vi "Butterfly_Resitance w_SMU.vi"(0 "Semiconductor Module Context":T3, 1 "script name":string="Cmax", 2 "SMU Settings":T2={"Level"=0.01, "Level Range"=0.1, "Limit"=1.0, "Limit Range"=6.0, "Sense"=0} {"Sense" items=["Local"=1008, "Remote"=1009]}, 5 "Pins":string[](array[string])=["RF"], 7 "HV_Voltages":dbl[](array[numeric]), 9 "Thresholds(max R 1st)":dbl[](array[numeric])=[100000.0, 0.5], 11 "error in (no error)":errorcluster) -> (4 "R Array":dbl[][](array[numeric]), 15 "error out":errorcluster)   [LabVIEW 2013]
uses:
  <vilib>/NI_TestStand_SemiconductorModule/NI_TestStand_Semiconductor_Module.lvlibp/PinMap/General/SemiconductorModuleContext.ctl
  <instrlib>/niDCPower/nidcpower.llb/niDCPower Sense.ctl
  <instrlib>/niHSDIO/niHSDIO.llb/niHSDIO_ctl Trigger Script - trigID Values (Ring).ctl
  <vilib>/NI_TestStand_SemiconductorModule/NI_TestStand_Semiconductor_Module.lvlibp/PinMap/General/Publish/PublishDataDoubleFunctionalTest.vi
  <vilib>/NI_TestStand_SemiconductorModule/NI_TestStand_Semiconductor_Module.lvlibp
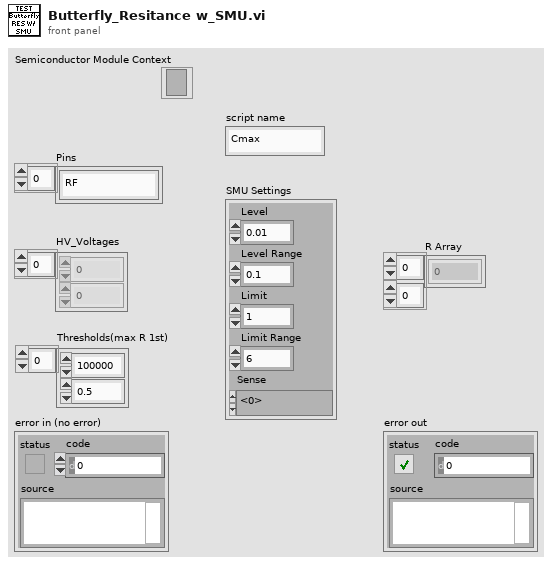
[diagram p1: front panel]
types:
  T1 = typedef "niDCPower Sense.ctl" = i32
  T2 = cluster{"Level":dbl, "Level Range":dbl, "Limit":dbl, "Limit Range":dbl, "Sense":T1}
  T3 = typedef "NI_TestStand_Semiconductor_Module.lvlibp/SemiconductorModuleContext.ctl" = refnum<k7>
  T4 = typedef "niHSDIO_ctl Trigger Script - trigID Values (Ring).ctl" = string
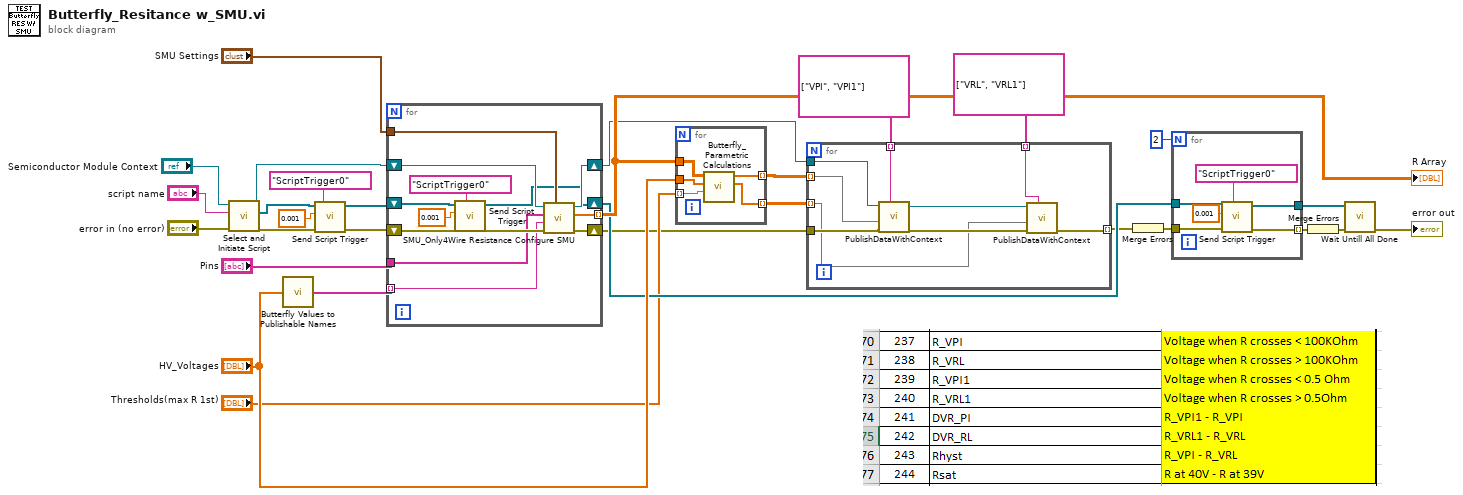
[diagram p0: block diagram]
diagram:
  n1 = call "Select and Initiate Script.vi"("error in (no error)"="error in (no error)", "script name"="script name", "Semiconductor Module Context"="Semiconductor Module Context") -> ("error out"=w6:errorcluster, "HSDIO GEN Sessions Out"=w3:refnum<k15>[], "Semiconductor Module Context Out"=w2:T3)  [unwired: 6 in]
  n2 = call "Butterfly Values to Publishable Names.vi"("Butterfly Numbers"="HV_Voltages") -> ("Publishable Names"=w27:string[])
  n3 = call "Send Script Trigger.vi"("trigger id (script trigger 0)"=T4 "ScriptTrigger0", "error in (no error)"=w6, "Delay Time (s)"=0.001, "HSDIO Sessions In"=w3) -> ("error out"=w5:errorcluster, "HSDIO Sessions Out"=w4:refnum<k15>[])  [unwired: 6 in]
  n4 = for {
    shift-right: [w40] -> w16
    shift-left: w5 -> [w43]
    shift-right: [w34] -> w15
    shift-left: w2 -> [w39]
    tunnel: w27 -> [w37] mode=indexing
    tunnel: "Pins" -> [w36]
    tunnel: "SMU Settings" -> [w35]
    tunnel: [w33] -> w23 mode=indexing
    shift-right: [w31] -> w20
    shift-left: w4 -> [w32]
    n5 = call "Send Script Trigger.vi"("trigger id (script trigger 0)"=T4 "ScriptTrigger0", "error in (no error)"=w43, "Delay Time (s)"=0.001, "HSDIO Sessions In"=w32) -> ("error out"=w41:errorcluster, "HSDIO Sessions Out"=w31:refnum<k15>[])  [unwired: 6 in]
    n6 = call "SMU_Only4Wire Resistance Configure SMU.vi"("SMU Settings"=w35, "error in (no error)"=w41, "Published Data Id"=w37, "Pins"=w36, "Semiconductor Module Context"=w39) -> ("error Out"=w40:errorcluster, "R Array"=w33:dbl[], "Semiconductor Module Context Out"=w34:T3)  [unwired: 4 in]
  }
  "R Array" <- w23
  n7 = for {
    tunnel: w23 -> [w48]
    tunnel: "HV_Voltages" -> [w47]
    tunnel: [w46] -> w12 mode=indexing
    tunnel: [w45] -> w11 mode=indexing
    tunnel: "Thresholds(max R 1st)" -> [w44] mode=indexing
    n8 = call "Butterfly_Parametric Calculations.vi"("Threshold"=w44, "Voltage Array"=w47, "Result Array In"=w48) -> ("VRLs"=w45:dbl[], "VPIs"=w46:dbl[])  [unwired: 7 in]
  }
  n9 = for {
    tunnel: w16 -> [w57]
    tunnel: w15 -> [w56]
    tunnel: [w54] -> w14 mode=indexing
    tunnel: w12 -> [w52] mode=indexing
    tunnel: w11 -> [w49] mode=indexing
    tunnel: string[] ["VPI", "VPI1"] -> [w51] mode=indexing
    tunnel: string[] ["VRL", "VRL1"] -> [w50] mode=indexing
    n10 = call-poly <vilib>:"PublishDataWithContext.vi"("Published Data Id"=w51, "error in (no error)"=w57, "Data In"=w52, "Semiconductor Module Context"=w56) -> ("error out"=w55:errorcluster, "Semiconductor Module Context Out"=w53:T3)  [unwired: 6 in]
    n11 = call-poly <vilib>:"PublishDataWithContext.vi"("Published Data Id"=w50, "error in (no error)"=w55, "Data In"=w49, "Semiconductor Module Context"=w53) -> ("error out"=w54:errorcluster)  [unwired: 6 in, 1 out]
  }
  n12 = Merge Errors(w14) -> (w13:errorcluster)
  n13 = for {
    N: 2 -> [_]
    tunnel: w20 -> [w63]
    tunnel: [w62] -> w19
    tunnel: [w61] -> w18 mode=indexing
    tunnel: w13 -> [w58]
    n14 = call "Send Script Trigger.vi"("trigger id (script trigger 0)"=T4 "ScriptTrigger0", "error in (no error)"=w58, "Delay Time (s)"=0.001, "HSDIO Sessions In"=w63) -> ("error out"=w61:errorcluster, "HSDIO Sessions Out"=w62:refnum<k15>[])  [unwired: 6 in]
  }
  n15 = Merge Errors(w18) -> (w21:errorcluster)
  n16 = call "Wait Untill All Done.vi"("error in (no error)"=w21, "HSDIO Sessions In"=w19) -> ("error out"=→"error out":errorcluster)  [unwired: 8 in, 1 out]
